vi "Get Size 1D.vi"(8 "error in (no error)":errorcluster, 11 "Const_I8_1D in":refnum<class "Const_U64_1D.lvclass">) -> (0 "error out":errorcluster, 2 "Size":i32, 3 "Const_I8_1D out":refnum<class "Const_U64_1D.lvclass">)   [LabVIEW 2021, in "Const_U64_1D.lvclass"]
uses:
  Const_U64_1D.lvclass
  Const_U64_1D.lvclass/Const_U64_1D.ctl
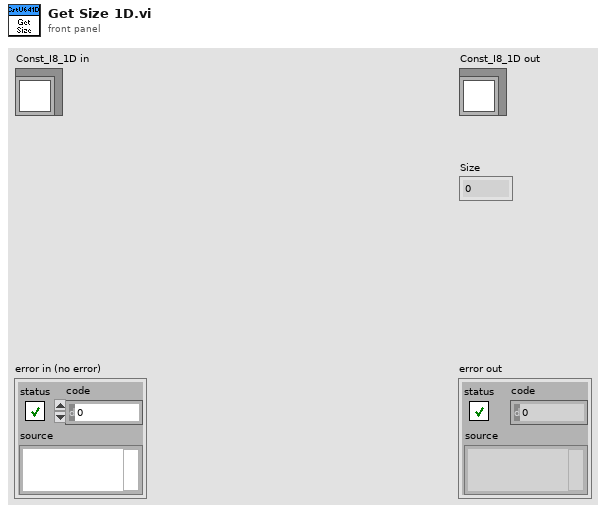
[diagram p1: front panel]
types:
  T1 = typedef "Const_U64_1D.lvclass/Type.ctl" = u64[]
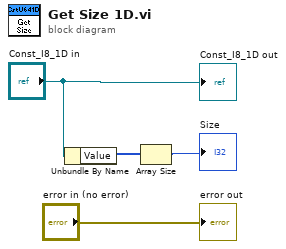
[diagram p0: block diagram]
diagram:
  n1 = Unbundle By Name("Const_I8_1D in") -> ("Value"=w2:T1)
  n2 = Array Size(array=w2) -> (size(s)=→"Size":i32)
  "error out" <- "error in (no error)"
  "Const_I8_1D out" <- "Const_I8_1D in"
